vi "init.vi"(0 "RS232-RTS High Test in":refnum<class "RS232-RTS High Test.lvclass">, 1 "MUX Settings":T1, 5 "ILC":refnum<class "ILC.lvclass">, 7 "ILC Digital Output Test":T3, 9 "Log":refnum<class "ITestLog.lvclass">, 11 "error in (no error)":errorcluster) -> (4 "RS232-RTS High Test out":refnum<class "RS232-RTS High Test.lvclass">, 15 "error out":errorcluster)   [LabVIEW 2015, in "RS232-RTS High Test.lvclass"]
uses:
  RS232-RTS High Test.lvclass
  <userlib>/Common/ilc/ILC/ILC.lvclass
  Typedefs/ILC Digital Output Test.ctl
  Typedefs/Digital Signal Level.ctl
  Model/TestLog/ITestLog/ITestLog.lvclass
  Typedefs/MUX Settings.ctl
  RS232-RTS High Test.lvclass/RS232-RTS High Test.ctl
  Typedefs/ILCBTTypedefs.lvlib
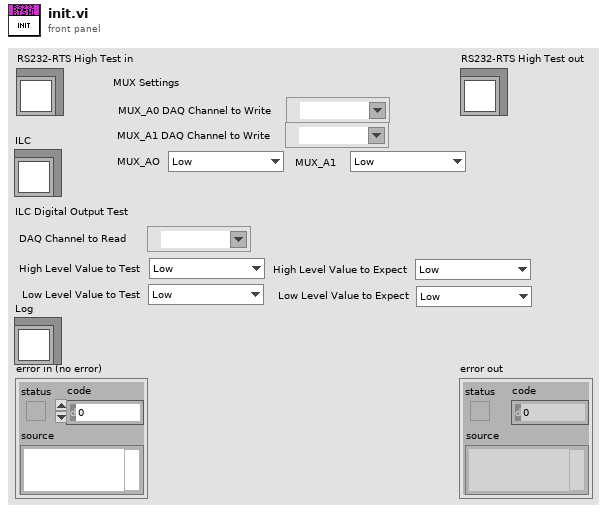
[diagram p1: front panel]
types:
  T1 = typedef "ILCBTTypedefs.lvlib/MUX Settings.ctl" = cluster{"MUX_AO":T2, "MUX_A1":T2, "MUX_A0 DAQ Channel to Write":refnum<k21>, "MUX_A1 DAQ Channel to Write":refnum<k21>}
  T2 = typedef "ILCBTTypedefs.lvlib/Digital Signal Level.ctl" = enum16{"Low", "High"}
  T3 = typedef "ILCBTTypedefs.lvlib/ILC Digital Output Test.ctl" = cluster{"DAQ Channel to Read":refnum<k21>, "High Level Value to Test":T2, "High Level Value to Expect":T2, "Low Level Value to Test":T2, "Low Level Value to Expect":T2}
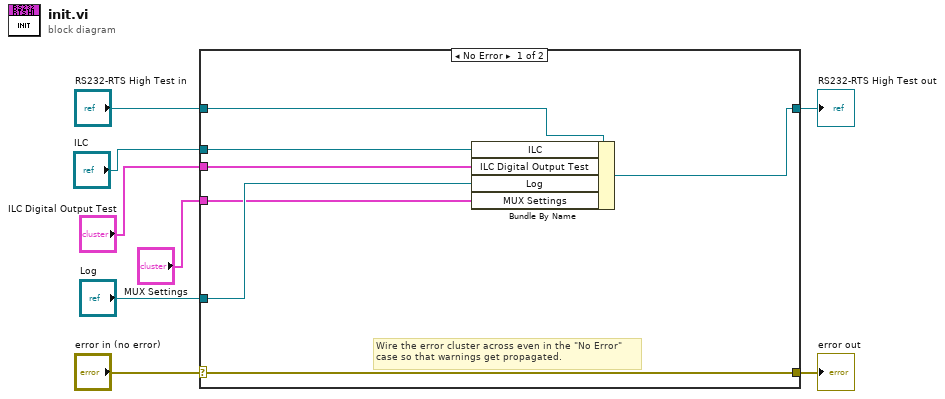
[diagram p0: block diagram]
diagram:
  n1 = case shown="No Error" "error in (no error)" {
    selector: "error in (no error)" -> [w15 w17]
    tunnel: [w15 w17] -> w7
    tunnel: [w13 w16] -> w5
    tunnel: "RS232-RTS High Test in" -> [w14 w16]
    tunnel: "ILC" -> [w12 _]
    tunnel: "ILC Digital Output Test" -> [w11 _]
    tunnel: "Log" -> [w10 _]
    tunnel: "MUX Settings" -> [w9 _]
    frame No Error {
      # "Wire the error cluster across even in the \"No Error\"\ncase so that warnings get propagated."
      n2 = Bundle By Name(cluster=w14, "ILC"=w12, "ILC Digital Output Test"=w11, "Log"=w10, "MUX Settings"=w9) -> (w13:refnum<class "RS232-RTS High Test.lvclass">)
    }
    frame Error {
    }
  }
  "error out" <- w7
  "RS232-RTS High Test out" <- w5
